vi "INCREMENT FILENAME v0.3.vi"(1 "FILENAME IN":string) -> (0 "FILENAME OUT":string)   [LabVIEW 2025]
doc: "Searches the filename for (XXXX.23) dot separator and a number following. If found, increments the number. If not, appends a dot and a one.\nScott Hannahs, FBNML, Feb 1992\nAuthor: Scott Hannahs <sth@magnet.fsu.edu>\n\nThis software is licensed for use under the “MIT License\"\nCopyright (c) 2025 Scott Hannahs, sth@sth@magnet.sthnet.net\n\nPermission is hereby granted, free of charge, to any person obtaining a copy of this software and associated documentation files (the \"Software\"), to deal in the Software without restriction, including without limitation the rights to use, copy, modify, merge, publish, distribute, sublicense, and/or sell copies of the Software, and to permit persons to whom the Software is furnished to do so, subject to the following conditions: The above copyright notice and this permission notice shall be included in all copies or substantial portions of the Software.\n\nTHE SOFTWARE IS PROVIDED \"AS IS\", WITHOUT WARRANTY OF ANY KIND, EXPRESS OR IMPLIED, INCLUDING BUT NOT LIMITED TO THE WARRANTIES OF MERCHANTABILITY, FITNESS FOR A PARTICULAR PURPOSE AND NONINFRINGEMENT. IN NO EVENT SHALL THE AUTHORS OR COPYRIGHT HOLDERS BE LIABLE FOR ANY CLAIM, DAMAGES OR OTHER LIABILITY, WHETHER IN AN ACTION OF CONTRACT, TORT OR OTHERWISE, ARISING FROM, OUT OF OR IN CONNECTION WITH THE SOFTWARE OR THE USE OR OTHER DEALINGS IN THE SOFTWARE."
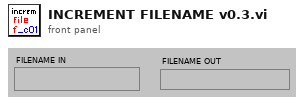
[diagram p1: front panel]
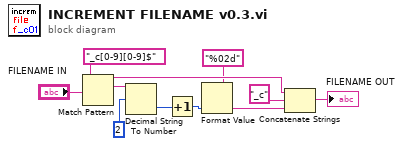
[diagram p0: block diagram]
diagram:
  n1 = Match Pattern(string="FILENAME IN", regular expression="_c[0-9][0-9]$") -> (before substring=w9:string, match substring=w7:string)  [unwired: 1 in, 2 out]
  n2 = Decimal String To Number(string=w7, offset=2) -> (number=w2:i32)  [unwired: 1 in, 1 out]
  n3 = Increment(x=w2) -> (x+1=w1:i32)
  n4 = Format Value(format string="%02d", value (0)=w1) -> (output string=w11:string)  [unwired: 1 in]
  n5 = Concatenate Strings(w9, "_c", w11) -> (→"FILENAME OUT":string)
